vi "calcCCmat.vi"(7 "zn3Idx":i32[](array[numeric]), 8 "error in (no error)":errorcluster, 9 "Effective Wavelength":dbl, 10 "PSSN Alpha":dbl[](array[numeric]), 11 "OptCtrl in":refnum<class "OptCtrl.lvclass">) -> (0 "error out":errorcluster, 2 "CC Matrix":dbl[][](array[numeric]), 3 "OptCtrl out":refnum<class "OptCtrl.lvclass">)   [LabVIEW 2016, in "OfcFunc.lvlib" / "OptCtrl.lvclass"]
doc: "Calculate the CC matrix used in matrix Q. It is C.T * C used in Q = A.T * (C.T * C) * A."
uses:
  OptCtrl.lvclass
  <vilib>/Analysis/7linalg.llb/Create Special Real Matrix.vi
  <vilib>/Analysis/Matrix/Numeric/Conversions/Matrix To Array - RM.vi
  MatOper/getSubArray2D.vi
  <vilib>/Analysis/NI_AALPro.lvlib
  <vilib>/Analysis/Matrix/NI_Matrix.lvlib
  MatOper/MatOper.lvclass
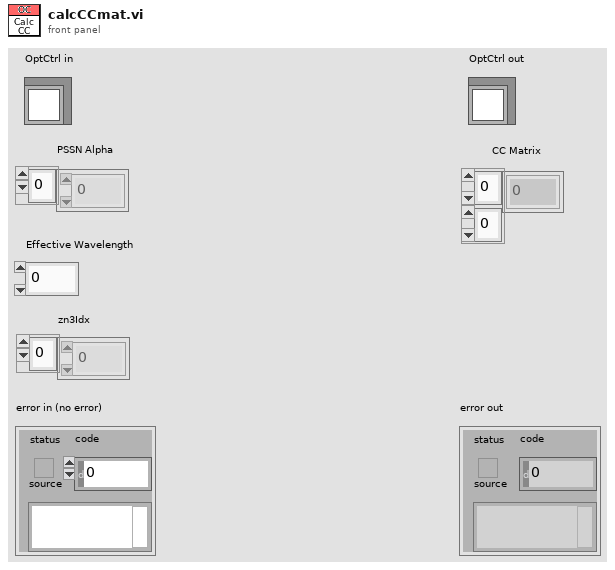
[diagram p1: front panel]
types:
  T1 = typedef "NI_Matrix.lvlib/RealMatrix.ctl" = dbl[][]
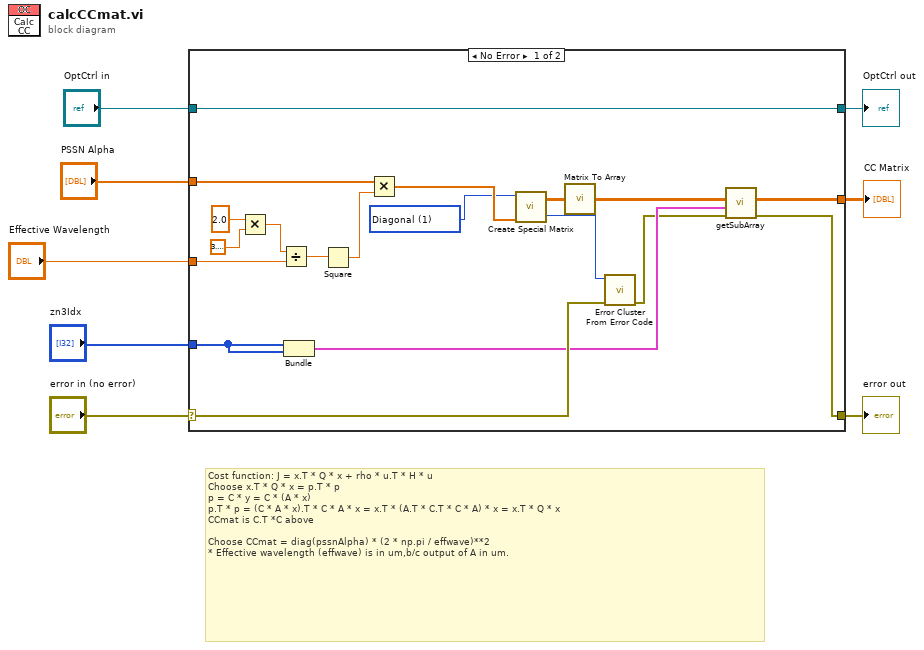
[diagram p0: block diagram]
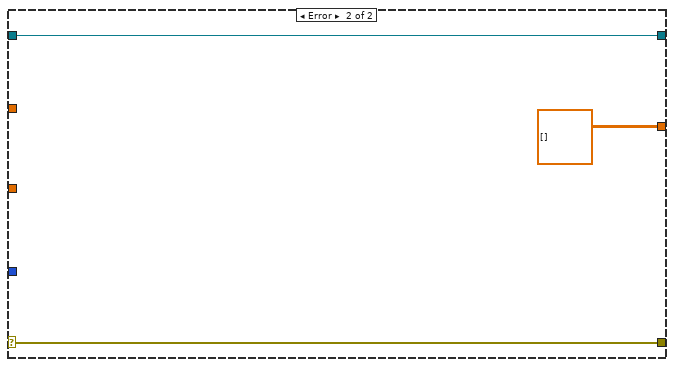
[diagram p2: hidden frame]
diagram:
  # "Cost function: J = x.T * Q * x + rho * u.T * H * u\nChoose x.T * Q * x = p.T * p\np = C * y = C * (A * x)\np.T * p = (C * A * x).T * C * A * x = x.T * (A.T * C.T * C * A) * x = x.T * Q * x\nCCmat is C.T *C above\n\nChoose CCmat = diag(pssnAlpha) * (2 * np.pi / effwave)**2\n* Effective wavelength (effwave) is in um,b/c output of A in um."
  n1 = case shown="No Error" "error in (no error)" {
    selector: "error in (no error)" -> [w16 w30]
    tunnel: [w10 w30] -> w7
    tunnel: [w27 w29] -> w5
    tunnel: "OptCtrl in" -> [w27 w29]
    tunnel: "Effective Wavelength" -> [w23 _]
    tunnel: "PSSN Alpha" -> [w21 _]
    tunnel: [w9 dbl[][] [] ("Real 2D Array")] -> w2
    tunnel: "zn3Idx" -> [w14 _]
    frame No Error {
      w18 = 1 items=["Identity", "Diagonal", "Toeplitz", "Vandermonde", "Companion", "Hankel", "Hadamard", "Wilkinson", "Hilbert", "Inverse Hilbert", "Rosser", "Pascal"] ("matrix type")
      n2 = Multiply(x=2.0, y=3.141592653589793) -> (x*y=w24:dbl)
      n3 = Divide(x=w24, y=w23) -> (x/y=w22:dbl)
      n4 = Bundle("zn3Idx"=w14, "zn3Idx"=w14) -> (w12:cluster{"zn3Idx":i32[], "zn3Idx":i32[]})  [unwired: 1 in]
      n5 = Square(x=w22) -> (x^2=w20:dbl)
      n6 = Multiply(x=w21, y=w20) -> (x*y=w19:dbl[])
      n7 = call-poly <vilib>:"Create Special Matrix.vi"("matrix type"=w18, "Input Vector1"=w19) -> ("Special Matrix"=w17:T1, "error"=w15:i32)  [unwired: 3 in]
      n8 = call-poly <vilib>:"Matrix To Array.vi"("Real Matrix"=w17) -> ("Real 2D Array"=w13:dbl[][])
      n9 = call <vilib>:"Error Cluster From Error Code.vi"("error in (no error)"=w16, "error code (0)"=w15) -> ("error out"=w11:errorcluster)  [unwired: 7 in]
      n10 = call-poly "getSubArray.vi"("error in (no error)"=w11, "Index Array Cluster"=w12, "2D Array"=w13) -> ("error out"=w10:errorcluster, "Sub-Array"=w9:dbl[][])  [unwired: 6 in, 1 out]
    }
    frame Error {
    }
  }
  "error out" <- w7
  "OptCtrl out" <- w5
  "CC Matrix" <- w2
